vi "Write Physical Camera Assignment.vi"(8 "error in (no error)":errorcluster, 10 "Array":T1[](array[typedef]), 11 "Camera in":refnum<class "Camera.lvclass">) -> (0 "error out":errorcluster, 3 "Camera out":refnum<class "Camera.lvclass">)   [LabVIEW 2018, in "Camera.lvlib" / "Camera.lvclass"]
uses:
  Camera.lvclass
  Resources/Type Defs/Physical Camera Assignment.ctl
  Resources/Type Defs/Camera Type.ctl
  Camera.lvclass/Camera.ctl
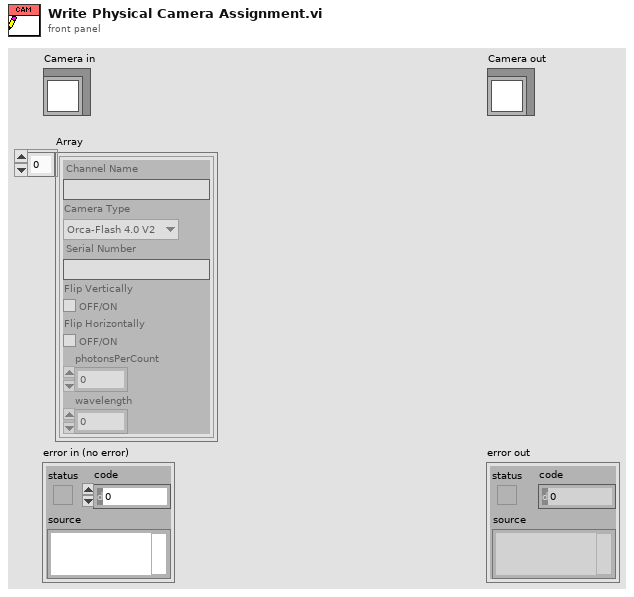
[diagram p1: front panel]
types:
  T1 = typedef "Physical Camera Assignment.ctl" = cluster{"Channel Name":string, "Camera Type":T2, "Serial Number":string, "Flip Vertically":bool, "Flip Horizontally":bool, "photonsPerCount":dbl, "wavelength":i16}
  T2 = typedef "Camera Type.ctl" = enum16{"Orca-Flash 4.0 V2"}
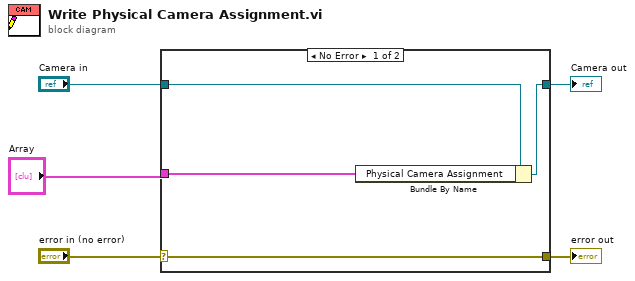
[diagram p0: block diagram]
diagram:
  n1 = case shown="No Error" "error in (no error)" {
    selector: "error in (no error)" -> [w9 w10]
    tunnel: [w9 w10] -> w4
    tunnel: [w7 w11] -> w2
    tunnel: "Camera in" -> [w8 w11]
    tunnel: "Array" -> [w6 _]
    frame No Error {
      n2 = Bundle By Name(cluster=w8, "Physical Camera Assignment"=w6) -> (w7:refnum<class "Camera.lvclass">)
    }
    frame Error {
    }
  }
  "error out" <- w4
  "Camera out" <- w2
